vi "HFRR ADV v025 new software.vi"() -> ()   [LabVIEW 2025] (continued)
                        n2432 = Number To Fractional String(number=w3641, precision (6)=i16 2) -> (F-format string=w3642:string)  [unwired: 2 in]
                        n2433 = Concatenate Strings("Set Stroke [mm] :" ("Content"), w3642) -> (w3644:string)
                        n2434 = local read "EVENT LOG"() -> (w3646:string)
                        n2435 = call "Event Log.vi"("Content"=w3644, "EVENT LOG"=w3646) -> ("EVENT LOG"=w3645:string)  [unwired: 8 in, 1 out]
                        n2436 = local write "EVENT LOG"(w3645) -> ()
                      }
                      frame #26 {
                        n2437 = Wait (ms)(milliseconds to wait=u32 50) -> ()  [unwired: 1 out]
                      }
                      frame #27 {
                        n2438 = local read "Set Temp"() -> (w3649:dbl)
                        n2439 = Number To Fractional String(number=w3649, precision (6)=i16 2) -> (F-format string=w3650:string)  [unwired: 2 in]
                        n2440 = Concatenate Strings("Set Temperature [deg C] :" ("Content"), w3650) -> (w3652:string)
                        n2441 = local read "EVENT LOG"() -> (w3654:string)
                        n2442 = call "Event Log.vi"("Content"=w3652, "EVENT LOG"=w3654) -> ("EVENT LOG"=w3653:string)  [unwired: 8 in, 1 out]
                        n2443 = local write "EVENT LOG"(w3653) -> ()
                      }
                      frame #28 {
                        n2444 = Wait (ms)(milliseconds to wait=u32 50) -> ()  [unwired: 1 out]
                      }
                      frame #29 {
                        n2445 = local read "Set Rh"() -> (w3657:dbl)
                        n2446 = Number To Fractional String(number=w3657, precision (6)=i16 2) -> (F-format string=w3658:string)  [unwired: 2 in]
                        n2447 = Concatenate Strings("Set Humidity [%RH] :" ("Content"), w3658) -> (w3660:string)
                        n2448 = local read "EVENT LOG"() -> (w3662:string)
                        n2449 = call "Event Log.vi"("Content"=w3660, "EVENT LOG"=w3662) -> ("EVENT LOG"=w3661:string)  [unwired: 8 in, 1 out]
                        n2450 = local write "EVENT LOG"(w3661) -> ()
                      }
                      frame #30 {
                        n2451 = Wait (ms)(milliseconds to wait=u32 50) -> ()  [unwired: 1 out]
                      }
                      frame #31 {
                        n2452 = local read "test time"() -> (w3665:dbl)
                        n2453 = Number To Fractional String(number=w3665, precision (6)=i16 1) -> (F-format string=w3666:string)  [unwired: 2 in]
                        n2454 = Concatenate Strings("Test Duration [mins] :" ("Content"), w3666) -> (w3668:string)
                        n2455 = local read "EVENT LOG"() -> (w3670:string)
                        n2456 = call "Event Log.vi"("Content"=w3668, "EVENT LOG"=w3670) -> ("EVENT LOG"=w3669:string)  [unwired: 8 in, 1 out]
                        n2457 = local write "EVENT LOG"(w3669) -> ()
                      }
                      frame #32 {
                        w3671 = dbl[] [] ("History Data")
                        w3672 = cluster{"y":dbl, dbl, "y":dbl}[] [] ("History Data")
                        w3673 = FALSE ("Visible")
                        n2458 = property on="Stroke ( mm )" class="WFChart (strict)"("History Data"=w3672) -> ()  [unwired: 2 in, 2 out]
                        n2459 = property on="Humidity ( %RH )" class="WFChart (strict)"("History Data"=w3671) -> ()  [unwired: 2 in, 2 out]
                        n2460 = property on="Temperature ( Deg C )" class="WFChart (strict)"("History Data"=w3671) -> ()  [unwired: 2 in, 2 out]
                        n2461 = property on="Electrical Contact Resistance ( % )" class="WFChart (strict)"("History Data"=w3671) -> ()  [unwired: 2 in, 2 out]
                        n2462 = property on="Coefficient of Friction" class="WFChart (strict)"("History Data"=w3671) -> ()  [unwired: 2 in, 2 out]
                        n2463 = property on="Frictional Force ( N )" class="WFChart (strict)"("History Data"=w3671) -> ()  [unwired: 2 in, 2 out]
                        n2464 = property on="Coefficient of Friction" class="WFChart (strict)"("History Data"=w3671) -> ()  [unwired: 2 in, 2 out]
                        n2465 = property on="Frictional Force ( N )" class="WFChart (strict)"("History Data"=w3671) -> ()  [unwired: 2 in, 2 out]
                        n2466 = property on="Electrical Contact Resistance ( % )" class="WFChart (strict)"("History Data"=w3671) -> ()  [unwired: 2 in, 2 out]
                        n2467 = property on="Humidity ( %RH )" class="WFChart (strict)"("History Data"=w3671) -> ()  [unwired: 2 in, 2 out]
                        n2468 = property on="Stroke ( mm )" class="WFChart (strict)"("History Data"=w3672) -> ()  [unwired: 2 in, 2 out]
                        n2469 = property on="Temperature ( Deg C )" class="WFChart (strict)"("History Data"=w3671) -> ()  [unwired: 2 in, 2 out]
                        n2470 = property on="Service Password Log" class="Str"("Visible"=w3673) -> ()  [unwired: 2 in, 2 out]
                        n2471 = property on="Password 3" class="Clust (strict)"("Visible"=w3673) -> ()  [unwired: 2 in, 2 out]
                      }
                    }
                    "TEST FILE NAM,E SAVED" <- TRUE ("TEST FILE NAM,E SAVED")
                  }
                }
              }
            }
          }
        }
        n2472 = case shown="True" w2970 {
          frame False {
            n2473 = local write "tfalg"(0.0 ("tfalg")) -> ()
          }
          frame True {
            n2474 = local read "tfalg"() -> (w3115:dbl)
            n2475 = Equal?(x=w3115, y=0.0) -> (x = y?=w3116:bool)
            n2476 = case shown="True" w3116 {
              frame False {
              }
              frame True {
                n2477 = local read "Total No. of Tests"() -> (w3119:dbl)
                n2478 = local write "tfalg"(1.0 ("tfalg")) -> ()
                n2479 = local write "acq 2"(FALSE ("acq 2")) -> ()
                n2480 = Wait (ms)(milliseconds to wait=u32 200) -> ()  [unwired: 1 out]
                n2481 = Increment(x=w3119) -> (x+1=w3118:dbl)
                n2482 = local write "Total No. of Tests"(w3118) -> ()
              }
            }
          }
        }
        n2483 = local write "Test \nStatus"(w2976) -> ()
        n2484 = local write "Save"(w2976) -> ()
        n2485 = local read "Main Tab"() -> (w2933:T2)
        n2486 = case shown="True" w2957 {
          tunnel: [FALSE ("RUN") TRUE ("RUN")] -> w2956
          tunnel: [_ 1] -> w2949
          frame False {
          }
          frame True {
          }
        }
        n2487 = In Range and Coerce(upper limit=w2964, x=w2937, lower limit=w2963) -> (In Range?=w2955:bool)  [unwired: 1 out]
        n2488 = In Range and Coerce(upper limit=w2961, x=w2936, lower limit=w2962) -> (In Range?=w2953:bool)  [unwired: 1 out]
        n2489 = case shown="True" w2969 {
          frame False {
            n2490 = local read "Rt 3"() -> (w3097:bool)
            n2491 = case shown="True" w3097 {
              frame False {
              }
              frame True {
                n2492 = local write "Rt 3"(FALSE ("Rt 3")) -> ()
                n2493 = local write "Json End Flg"(TRUE ("Upld AR 2")) -> ()
              }
            }
            "Rt" <- TRUE ("Rt")
            "Rt 2" <- FALSE ("Rt")
          }
          frame True {
            n2494 = local read "Rt"() -> (w3104:bool)
            n2495 = local write "Rt 2"(TRUE ("Rt 2")) -> ()
            n2496 = case shown="True" w3104 {
              frame False {
              }
              frame True {
                w3105 = TRUE ("Upld AR 2")
                n2497 = local write "Rt"(FALSE ("Rt")) -> ()
                n2498 = local write "Upld AR"(w3105) -> ()
                n2499 = local write "Json St Flg"(w3105) -> ()
              }
            }
            "Rt 3" <- TRUE ("Rt 3")
          }
        }
        n2500 = case shown="True" w2955 {
          tunnel: [FALSE ("RUN") TRUE ("RUN")] -> w2954
          tunnel: [_ 2] -> w2948
          frame False {
          }
          frame True {
          }
        }
        n2501 = case shown="True" w2953 {
          tunnel: [FALSE ("RUN") TRUE ("RUN")] -> w2952
          tunnel: [_ 3] -> w2947
          frame False {
          }
          frame True {
          }
        }
        n2502 = case shown="\"Acquire\"" w2933 {
          tunnel: w2935 -> [_ w3166]
          frame Default {
            w3165 = 0.0 ("output")
            n2503 = local write "PID-out"(w3165) -> ()
            n2504 = local write "Frequency ( Hz )"(w3165) -> ()
          }
          frame "Acquire" {
            n2505 = stacked-sequence {
              frame #0 {
                n2506 = local read "Auto Start Test"() -> (w3168:bool)
                n2507 = case shown="True" w3168 {
                  tunnel: "RUN" -> [w3189 w3192]
                  tunnel: [w3189 w3191] -> w3169
                  frame False {
                  }
                  frame True {
                    n2508 = local read "Auto Start Temp"() -> (w3190:bool)
                    n2509 = Or(x=w3192, y=w3190) -> (x .or. y?=w3191:bool)
                  }
                }
                n2510 = local read "clk"() -> (w3188:dbl)
                n2511 = local read "Save"() -> (w3184:bool)
                n2512 = Equal?(x=w3188, y=0.0) -> (x = y?=w3185:bool)
                n2513 = And(x=w3185, y=w3184) -> (x .and. y?=w3186:bool)
                n2514 = Not(x="Engage") -> (.not. x?=w3175:bool)
                n2515 = case shown="False" w3169 {
                  tunnel: [0.0 w3215] -> w3171
                  frame False {
                    (unwired) TRUE ("Visible")
                    n2516 = local read "Auto Start Test"() -> (w3196:bool)
                    n2517 = local write "Start Time"(TRUE ("Start Time")) -> ()
                    n2518 = property on="Stroke 2" class="DigNum (strict)"("Visible"=FALSE) -> ()  [unwired: 2 in, 2 out]
                    n2519 = case shown="False" w3196 {
                      frame False {
                        n2520 = property on="Heater Button" class="Bool (strict)"("DisabledEnum"=T17."Enabled" ("Disabled")) -> ()  [unwired: 2 in, 2 out]
                        n2521 = property on="Humidity" class="Bool (strict)"("DisabledEnum"=T17."Enabled" ("Disabled")) -> ()  [unwired: 2 in, 2 out]
                      }
                      frame True {
                      }
                    }
                    n2522 = case shown="False" "TestCompFlg" {
                      frame False {
                        n2523 = local read "StartFlg"() -> (w3204:bool)
                        n2524 = case shown="True" w3204 {
                          frame False {
                          }
                          frame True {
                            n2525 = stacked-sequence {
                              frame #0 {
                                n2526 = local read "EVENT LOG"() -> (w3208:string)
                                n2527 = call "Event Log.vi"("Content"="Test was interrupted", "EVENT LOG"=w3208) -> ("EVENT LOG"=w3209:string)  [unwired: 8 in, 1 out]
                                n2528 = local write "EVENT LOG"(w3209) -> ()
                                n2529 = property on="RUN" class="Bool (strict)"("Visible"=TRUE) -> ()  [unwired: 2 in, 2 out]
                                n2530 = property on="Auto Start Test" class="Bool (strict)"("Visible"=TRUE) -> ()  [unwired: 2 in, 2 out]
                              }
                              frame #1 {
                                w3211 = FALSE ("StartFlg")
                                n2531 = property on="Heater Button" class="Bool (strict)"("Val(Sgnl)"=FALSE ("Value (Signaling)")) -> ()  [unwired: 2 in, 2 out]
                                n2532 = local write "Heater Button"(w3211) -> ()
                                n2533 = local write "StartFlg"(w3211) -> ()
                                n2534 = local write "Humidity"(w3211) -> ()
                              }
                              frame #2 {
                                n2535 = local write "Due Write"("VC;0" ("Command")) -> ()
                              }
                              frame #3 {
                                n2536 = Wait (ms)(milliseconds to wait=u32 1500) -> ()  [unwired: 1 out]
                              }
                              frame #4 {
                                n2537 = local write "Due Write"("HE;0" ("Command")) -> ()
                              }
                            }
                          }
                        }
                      }
                      frame True {
                      }
                    }
                    n2538 = local write "String 14"("Test will autostart once parameters reach the set value." ("String 14")) -> ()
                  }
                  frame True {
                    (unwired) FALSE ("Visible")
                    n2539 = property on="Stroke 2" class="DigNum (strict)"("Visible"=TRUE) -> ()  [unwired: 2 in, 2 out]
                    n2540 = property on="STOP 2" class="Bool (strict)"("Disabled"=u8 2) -> ()  [unwired: 2 in, 2 out]
                    n2541 = local write "String 14"(" Running....." ("String 14")) -> ()
                    n2542 = property on="Heater Button" class="Bool (strict)"("DisabledEnum"=T17."Disabled and Grayed Out" ("Disabled")) -> ()  [unwired: 2 in, 2 out]
                    n2543 = property on="Humidity" class="Bool (strict)"("DisabledEnum"=T17."Disabled and Grayed Out" ("Disabled")) -> ()  [unwired: 2 in, 2 out]
                    n2544 = case shown="True" "Start Time" {
                      selector: "Start Time" -> [_ w3234]
                      frame False {
                      }
                      frame True {
                        n2545 = Not(x=w3234) -> (.not. x?=w3233:bool)
                        n2546 = local write "Start Time"(w3233) -> ()
                        n2547 = local read "EVENT LOG"() -> (w3235:string)
                        n2548 = call "Event Log.vi"("Content"="Test in progress", "EVENT LOG"=w3235) -> ("EVENT LOG"=w3237:string)  [unwired: 8 in, 1 out]
                        n2549 = local write "EVENT LOG"(w3237) -> ()
                      }
                    }
                    n2550 = disable-structure shown="Enabled" {
                      disable-tunnel: [w3226 w3232] -> w3215
                      frame Disabled {
                        n2551 = local read "Set Hz"() -> (w3229:dbl)
                        n2552 = call <vilib>:"Uniform White Noise Waveform.vi"() -> ("signal out"=w3228:waveform(dbl))  [unwired: 10 in, 1 out]
                        n2553 = Random Number (0-1)() -> (number: 0 to 1=w3225:dbl)
                        n2554 = Add(x=w3229, y=w3228) -> (x+y=w3227:waveform(dbl))
                        n2555 = Multiply(x=ext 0.01 ("y"), y=w3225) -> (x*y=w3223:ext)
                        n2556 = Multiply(x=w3227, y=w3223) -> (x*y=w3226:waveform(ext))
                      }
                      frame Enabled {
                        n2557 = call-poly <vilib>:"Random Number (Range).vi"("lower bound (0)"=49.89, "upper bound (100)"=50.8) -> ("number"=w3232:dbl)  [unwired: 9 in]
                      }
                    }
                    "StartFlg" <- TRUE ("StartFlg")
                  }
                }
                n2558 = case shown="True" w3186 {
                  frame False {
                  }
                  frame True {
                    n2559 = local write "clk"(10.0 ("clk")) -> ()
                    n2560 = Get Date/Time In Seconds() -> (seconds since 1Jan1904=w3240:timestamp)
                    n2561 = To Double Precision Float(number=w3240) -> (double precision float=w3238:dbl)
                    n2562 = local write "acq timer"(w3238) -> ()
                    n2563 = local write "act save time"(w3238) -> ()
                  }
                }
                n2564 = call "Elapsed Time"("Time Target (s)"="Countdown", "Reset"=w3175) -> ("Elapsed Time (s)"=w3180:dbl, "Time has Elapsed"=w3178:bool)  [unwired: 10 in, 6 out]
                "Countdown 2" <- w3180
                n2565 = Subtract(x=w3180, y=2.0) -> (x-y=w3183:dbl)
                n2566 = Less?(x=w3183, y="Countdown") -> (x < y?=w3181:bool)
                n2567 = And(x=w3181, y=w3178) -> (x .and. y?=w3177:bool)
                n2568 = case shown="True" w3177 {
                  frame False {
                  }
                  frame True {
                    (unwired) dbl[] [] ("History Data")
                    n2569 = local write "Engage"(FALSE ("Engage")) -> ()
                    n2570 = local write "RUN"(TRUE ("RUN")) -> ()
                    n2571 = local read "Humidity ( %RH )"() -> (→"Rh Before":dbl)
                  }
                }
                n2572 = local read "Test \nStatus"() -> (w3173:bool)
                n2573 = Select(t=w3171, s=w3173, f=0.0) -> (s? t:f=w3172:dbl)
                n2574 = local write "Frequency ( Hz )"(w3172) -> ()
              }
              frame #1 {
                w3263 = 1000000.0 ("x")
                # "HC;1/0\nST;VALUE"
                # "Elapsed time\ncof\nstroke\nAir temp\nTemp\nHumidity"
                # "acq timer\n\nact save time"
                # "convert to microseconds"
                n2575 = local read "COUNT"() -> (w3246:i32)
                n2576 = local read "Rate"() -> (w3259:dbl)
                n2577 = Divide(x=w3263, y=w3259) -> (x/y=w3264:dbl)
                n2578 = Greater Or Equal?(x=w3246, y=250) -> (x >= y?=w3245:bool)
                n2579 = Get Date/Time In Seconds() -> (seconds since 1Jan1904=w3266:timestamp)
                n2580 = case shown="True" w3245 {
                  frame False {
                    n2581 = local read "COUNT"() -> (w3267:i32)
                    n2582 = Increment(x=w3267) -> (x+1=w3268:i32)
                    n2583 = local write "COUNT"(w3268) -> ()
                  }
                  frame True {
                    n2584 = local write "COUNT"(0 ("COUNT")) -> ()
                  }
                }
                n2585 = local read "Samplingtime 2"() -> (w3244:dbl)
                n2586 = local read "act save time"() -> (w3261:dbl)
                n2587 = Divide(x=w3264, y=w3263) -> (x/y=w3262:dbl)
                n2588 = To Double Precision Float(number=w3266) -> (double precision float=w3255:dbl)
                n2589 = Add(x=w3261, y=w3244) -> (x+y=w3260:dbl)
                n2590 = local read "acq timer"() -> (w3265:dbl)
                n2591 = local read "COUNT"() -> (w3248:i32)
                n2592 = Greater Or Equal?(x=w3255, y=w3260) -> (x >= y?=w3243:bool)
                n2593 = Multiply(x=w3262, y=w3248) -> (x*y=w3254:dbl)
                n2594 = Subtract(x=w3255, y=w3265) -> (x-y=w3257:dbl)
                n2595 = local read "Save"() -> (w3258:bool)
                n2596 = Add(x=w3257, y=w3254) -> (x+y=w3241:dbl)
                "Elapsed time 3" <- w3241
                n2597 = And(x=w3243, y=w3258) -> (x .and. y?=w3256:bool)
                n2598 = Divide(x=w3241, y=60.0) -> (x/y=w3252:dbl)
                n2599 = local read "Test \nStatus"() -> (w3242:bool)
                n2600 = local read "clk"() -> (w3249:dbl)
                n2601 = Equal?(x=w3249, y=10.0) -> (x = y?=w3251:bool)
                n2602 = case shown="True" w3256 {
                  tunnel: w3255 -> [_ w3379]
                  tunnel: [FALSE ("Boolean 2") TRUE ("Boolean 2")] -> _
                  frame False {
                  }
                  frame True {
                    w3333 = ";" ("Substring")
                    # "Pid out/\nFreq response value"
                    n2603 = local write "act save time"(w3379) -> ()
                    n2604 = local read "FILE"() -> (w3327:string)
                    n2605 = call "file check.vi"("file name in"=w3327) -> ("error out"=w3330:errorcluster, "file name out"=w3325:string)  [unwired: 9 in]
                    n2606 = local read "LVDT STROKE"() -> (w3322:dbl)
                    n2607 = local read "Add up Stroke"() -> (w3320:dbl)
                    n2608 = call "FILE PATH CREATION.vi"("error in"=w3330, "FILE NAME :"=w3325) -> ("FILE OUT"=w3328:path)  [unwired: 8 in, 1 out]
                    n2609 = Concatenate Strings(w3325, ".dgf" ("Substring")) -> (w3329:string)
                    n2610 = Subtract(x=w3322, y=w3320) -> (x-y=w3321:dbl)
                    n2611 = Absolute Value(x=w3321) -> (abs(x)=w3319:dbl)
                    n2612 = local read "FF 2"() -> (→"Frictional Force ( N )" →"Frictional Force ( N )":dbl)
                    n2613 = Build Path(base path=w3328, name or relative path=w3329) -> (appended path=w3324:path)
                    n2614 = local read "COF 2"() -> (w3338:dbl)
                    "cof" <- w3338
                    "Coefficient of Friction" <- w3338
                    "COF 4" <- w3338
                    "Coefficient of Friction" <- w3338
                    n2615 = local read "TEMP"() -> (w3341:dbl)
                    "Temp" <- w3341
                    "Temperature ( Deg C )" <- w3341
                    n2616 = local read "Humidity ( %RH )"() -> (w3340:dbl)
                    "Humidity ( %RH )" <- w3340
                    "Humidity ( %RH )" <- w3340
                    n2617 = local read "Frequency ( Hz )"() -> (w3347:dbl)
                    n2618 = call <vilib>:"Mean PtByPt.vi"("x"=w3319, "sample length"="STROKE FILTER") -> ("mean"=w3318:dbl)  [unwired: 2 in, 1 out]
                    n2619 = local read "Elapsed time"() -> (w3372:dbl)
                    n2620 = local read "AIR TEMP"() -> (w3345:dbl)
                    n2621 = local read "PID-out"() -> (w3350:dbl)
                    n2622 = local write "Temperature ( Deg C )"(w3341) -> ()
                    n2623 = Number To Fractional String(number=w3318, width (-)=i16 9 ("precision (6)"), precision (6)=i16 6) -> (F-format string=w3365:string)  [unwired: 1 in]
                    n2624 = Number To Fractional String(number=w3345, width (-)=i16 9 ("precision (6)"), precision (6)=i16 3) -> (F-format string=w3364:string)  [unwired: 1 in]
                    n2625 = Number To Fractional String(number=w3341, width (-)=i16 9 ("precision (6)"), precision (6)=i16 3) -> (F-format string=w3361:string)  [unwired: 1 in]
                    n2626 = Number To Fractional String(number=w3340, width (-)=i16 9 ("precision (6)"), precision (6)=i16 3) -> (F-format string=w3358:string)  [unwired: 1 in]
                    n2627 = Number To Fractional String(number=0.0, width (-)=i16 9 ("precision (6)"), precision (6)=i16 3) -> (F-format string=w3355:string)  [unwired: 1 in]
                    n2628 = Number To Fractional String(number=w3350, width (-)=i16 9 ("precision (6)"), precision (6)=i16 3) -> (F-format string=w3351:string)  [unwired: 1 in]
                    n2629 = Number To Fractional String(number=w3347, width (-)=i16 9 ("precision (6)"), precision (6)=i16 3) -> (F-format string=w3346:string)  [unwired: 1 in]
                    n2630 = Number To Fractional String(number=w3338, width (-)=i16 9 ("precision (6)"), precision (6)=i16 6) -> (F-format string=w3373:string)  [unwired: 1 in]
                    n2631 = Number To Fractional String(number=w3372, width (-)=i16 14 ("precision (6)"), precision (6)=i16 3) -> (F-format string=w3374:string)  [unwired: 1 in]
                    n2632 = Bundle("y"=1.02, "mean"=w3318, "y"=0.98) -> (w3339:cluster{"y":dbl, "mean":dbl, "y":dbl})  [unwired: 1 in]
                    n2633 = Number To Fractional String(number="Ambient Humidity :", width (-)=i16 9 ("precision (6)"), precision (6)=i16 6) -> (F-format string=w3331:string)  [unwired: 1 in]
                    n2634 = local read "RUN"() -> (w3337:bool)
                    n2635 = case shown="True" w3337 {
                      tunnel: w3339 -> [_ w3384]
                      tunnel: w3318 -> [_ w3383]
                      tunnel: w3318 -> [_ w3381]
                      tunnel: w3318 -> [_ w3382]
                      frame False {
                      }
                      frame True {
                        "Stroke ( mm )" <- w3384
                        "Stroke ( mm )" <- w3384
                        "Stroke 4" <- w3383
                        "Stroke 3" <- w3381
                        "Stroke 2" <- w3382
                        "measured_stroke" <- w3381
                      }
                    }
                    n2636 = Concatenate Strings(w3374, w3333, w3373, w3333, w3365, w3333, w3364, w3333, w3361, w3333, w3358, w3333, w3355, w3333, w3351, w3333, w3346, w3333, w3331, "\r") -> (w3371:string)
                    n2637 = call <vilib>:"Write Characters To File.vi"("append to file? (new file:F)"=TRUE, "character string"=w3371, "file path (dialog if empty)"=w3324) -> ()  [unwired: 2 in, 1 out]
                    "refresh flag" <- TRUE ("refresh flag")
                  }
                }
                n2638 = case shown="True" w3242 {
                  tunnel: w3252 -> [_ w3278]
                  tunnel: w3257 -> [_ w3288]
                  tunnel: [0.0 w3284] -> _
                  tunnel: w3251 -> [_ w3283]
                  tunnel: [0.0 w3282] -> _
                  tunnel: w3241 -> [_ w3282]
                  tunnel: w3255 -> [w3271 _]
                  frame False {
                    n2639 = local write "acq timer"(w3271) -> ()
                    n2640 = local write "Test Duration Status"(0.0 ("Test Duration Status")) -> ()
                  }
                  frame True {
                    n2641 = local read "Set Hz"() -> (w3285:dbl)
                    n2642 = local write "Elapsed time"(w3278) -> ()
                    n2643 = local read "test time"() -> (w3277:dbl)
                    n2644 = Multiply(x=w3288, y=w3285) -> (x*y=w3287:dbl)
                    n2645 = case shown="False" w3283 {
                      tunnel: w3287 -> [w3289 _]
                      tunnel: [w3289 1.0] -> w3284
                      frame False {
                        n2646 = local write "Cycles elapsed"(w3289) -> ()
                      }
                      frame True {
                      }
                    }
                    n2647 = Greater?(x=w3278, y=w3277) -> (0:w3286:bool)
                    n2648 = Subtract(x=w3277, y=w3278) -> (x-y=w3276:dbl)
                    "time" <- w3276
                    n2649 = Multiply(x=w3276, y=60.0) -> (x*y=w3275:dbl)
                    n2650 = local write "Time Remaining"(w3275) -> ()
                    n2651 = local write "Remaining Time"(w3275) -> ()
                    n2652 = case shown="True" w3286 {
                      frame False {
                      }
                      frame True {
                        n2653 = stacked-sequence {
                          frame #0 {
                            w3294 = T17."Enabled" ("Disabled")
                            w3293 = FALSE ("TEST FILE NAM,E SAVED")
                            w3295 = "" ("FILE")
                            w3296 = TRUE ("Visible")
                            n2654 = local write "Humidity"(FALSE ("Humidity")) -> ()
                            n2655 = local write "RUN"(FALSE ("OK Button 2")) -> ()
                            n2656 = local write "Heater Button"(FALSE ("Heater Button")) -> ()
                            n2657 = local write "Auto Start Test"(FALSE ("Auto Start Test")) -> ()
                            n2658 = local write "TestCompFlg"(TRUE ("StpFlg")) -> ()
                            n2659 = local read "Humidity ( %RH )"() -> (→"Rh After":dbl)
                            n2660 = property on="STOP 2" class="Bool (strict)"("Disabled"=u8 0) -> ()  [unwired: 2 in, 2 out]
                            n2661 = local read "EVENT LOG"() -> (w3301:string)
                            n2662 = call "Event Log.vi"("Content"="Test Completed", "EVENT LOG"=w3301) -> ("EVENT LOG"=w3300:string)  [unwired: 8 in, 1 out]
                            n2663 = property on="RUN" class="Bool (strict)"("Visible"=w3296) -> ()  [unwired: 2 in, 2 out]
                            n2664 = property on="Auto Start Test" class="Bool (strict)"("Visible"=w3296) -> ()  [unwired: 2 in, 2 out]
                            n2665 = local write "Batch Ref Num :"(w3295) -> ()
                            n2666 = local write "FILE"(w3295) -> ()
                            n2667 = local write "EVENT LOG"(w3300) -> ()
                            n2668 = local write "TEST FILE NAM,E SAVED"(w3293) -> ()
                            n2669 = local write "Fuel Discription :"(w3295) -> ()
                            n2670 = local write "START TEMP"(w3293) -> ()
                            n2671 = local write "Remarks :"(w3295) -> ()
                            n2672 = local write "Main Dashboard Buttons"(T1."Imaging" ("Main Dashboard Buttons")) -> ()
                            n2673 = local write "Main Tab"(T2."Adv Scar" ("Main Tab")) -> ()
                            n2674 = property on="FRICVALZ 2" class="Bool (strict)"("DisabledEnum"=w3294) -> ()  [unwired: 2 in, 2 out]
                            n2675 = property on="FRICVALZ 3" class="Bool (strict)"("DisabledEnum"=w3294) -> ()  [unwired: 2 in, 2 out]
                            n2676 = property on="FRICVALZ 4" class="Bool (strict)"("DisabledEnum"=w3294) -> ()  [unwired: 2 in, 2 out]
                          }
                          frame #1 {
                            n2677 = Wait (ms)(milliseconds to wait=u32 1500) -> ()  [unwired: 1 out]
                          }
                          frame #2 {
                            n2678 = local write "Due Write"("VC;0") -> ()
                          }
                          frame #3 {
                            n2679 = Wait (ms)(milliseconds to wait=u32 1500) -> ()  [unwired: 1 out]
                          }
                          frame #4 {
                            n2680 = local write "Due Write"("VC;0") -> ()
                          }
                          frame #5 {
                            n2681 = Wait (ms)(milliseconds to wait=u32 1500) -> ()  [unwired: 1 out]
                          }
                          frame #6 {
                            n2682 = local write "Due Write"("ST;0") -> ()
                          }
                          frame #7 {
                            n2683 = local write "measured_stroke"(0.0 ("measured_stroke")) -> ()
                            n2684 = Wait (ms)(milliseconds to wait=u32 1500) -> ()  [unwired: 1 out]
                          }
                          frame #8 {
                            n2685 = local write "Due Write"("HE;0") -> ()
                          }
                        }
                      }
                    }
                    n2686 = Divide(x=w3278, y=w3277) -> (x/y=w3281:dbl)
                    n2687 = Multiply(x=w3281, y=100.0) -> (x*y=w3279:dbl)
                    n2688 = local write "Test Duration Status"(w3279) -> ()
                  }
                }
              }
              frame #2 {
                n2689 = case shown="True" "Heater Button" {
                  tunnel: [0.0 ("output") w3407] -> w3385
                  frame False {
                    w3388 = TRUE ("tmpchk")
                    n2690 = local read "TEMP"() -> (w3389:dbl)
                    n2691 = local write "Temp ini"(w3389) -> ()
                    n2692 = local write "Reset 4"(w3388) -> ()
                    n2693 = local write "tmpchk"(w3388) -> ()
                    n2694 = local write "reinit"(TRUE ("reinit")) -> ()
                    n2695 = local write "manual temp log"(TRUE ("manual temp log")) -> ()
                  }
                  frame True {
                    # "Logic to turn off\nthe heater when \ntemp is not rising.\nTime - 60 sec\nDelta t- 5°c"
                    n2696 = local read "Temp ini"() -> (w3396:dbl)
                    n2697 = local read "Auto Start Test"() -> (w3392:bool)
                    n2698 = Less?(x=w3396, y=53.0) -> (x < y?=w3394:bool)
                    n2699 = case shown="False" w3392 {
                      frame False {
                        n2700 = local read "Set Temp"() -> (w3416:dbl)
                        n2701 = local read "TEMP"() -> (w3415:dbl)
                        n2702 = Subtract(x=w3416, y=w3415) -> (x-y=w3414:dbl)
                        n2703 = Absolute Value(x=w3414) -> (abs(x)=w3413:dbl)
                        n2704 = Less?(x=w3413, y=0.5) -> (x < y?=w3411:bool)
                        n2705 = case shown="True" w3411 {
                          tunnel: "manual temp log" -> [_ w3417]
                          frame False {
                          }
                          frame True {
                            n2706 = case shown="True" w3417 {
                              selector: w3417 -> [_ w3418]
                              frame False {
                              }
                              frame True {
                                # "#Event log"
                                n2707 = Not(x=w3418) -> (.not. x?=w3419:bool)
                                n2708 = local write "manual temp log"(w3419) -> ()
                                n2709 = local read "EVENT LOG"() -> (w3422:string)
                                n2710 = call "Event Log.vi"("Content"="Target Temperature reached", "EVENT LOG"=w3422) -> ("EVENT LOG"=w3421:string)  [unwired: 8 in, 1 out]
                                n2711 = local write "EVENT LOG"(w3421) -> ()
                              }
                            }
                          }
                        }
                      }
                      frame True {
                        n2712 = local write "manual temp log"(TRUE ("manual temp log")) -> ()
                      }
                    }
                    n2713 = And(x="tmpchk", y=w3394) -> (x .and. y?=w3397:bool)
                    n2714 = case shown="True" w3397 {
                      frame False {
                      }
                      frame True {
                        n2715 = call "Elapsed Time8"("Time Target (s)"=300.0, "Reset"="Reset 4") -> ("Time has Elapsed"=w3424:bool)  [unwired: 10 in, 7 out]
                        n2716 = flat-sequence {
                          tunnel: w3424 -> [_]
                          frame #0 {
                            n2717 = local write "Reset 4"(FALSE ("Reset 4")) -> ()
                          }
                        }
                        n2718 = case shown="True" w3424 {
                          frame False {
                          }
                          frame True {
                            n2719 = local read "Temp ini"() -> (w3431:dbl)
                            n2720 = Add(x=w3431, y=5.0) -> (x+y=w3429:dbl)
                            n2721 = local read "TEMP"() -> (w3432:dbl)
                            n2722 = Greater?(x=w3432, y=w3429) -> (0:w3430:bool)
                            n2723 = case shown="False" w3430 {
                              frame False {
                                n2724 = local write "Heater Button"(FALSE ("Heater Button")) -> ()
                              }
                              frame True {
                                n2725 = local write "tmpchk"(FALSE ("tmpchk")) -> ()
                              }
                            }
                          }
                        }
                      }
                    }
                    n2726 = local read "Set Temp"() -> (w3405:dbl)
                    n2727 = local read "TEMP"() -> (w3399:dbl)
                    n2728 = call-poly <vilib>:"PID.vi"("reinitialize? (F)"="reinit", "dt (s)"=-1.0, "process variable"=w3399, "setpoint"=w3405) -> ("output"=w3402:dbl)  [unwired: 6 in, 1 out]
                    n2729 = Subtract(x=w3405, y=w3399) -> (x-y=w3406:dbl)
                    n2730 = Add(x=w3405, y=0.5) -> (x+y=w3403:dbl)
                    n2731 = Greater Or Equal?(x=w3399, y=w3403) -> ()  [unwired: 1 out]
                    n2732 = Select(t=0.0, s=FALSE, f=w3402) -> (s? t:f=w3401:dbl)
                    "PID output" <- w3401
                    n2733 = flat-sequence {
                      tunnel: w3401 -> [w3435]
                      tunnel: [w3435] -> w3407
                      frame #0 {
                        n2734 = local write "reinit"(FALSE ("reinit")) -> ()
                      }
                    }
                    n2735 = Bundle(w3406, "output"=w3401, "TEMP"=w3399) -> ()  [unwired: 1 in, 1 out]
                  }
                }
                "PID-out" <- w3385
              }
              frame #3 {
                n2736 = local read "TEMP"() -> (w3437:dbl)
                n2737 = Greater Or Equal?(x=w3437, y="Set Temp 2") -> (x >= y?=w3442:bool)
                n2738 = case shown="True" w3442 {
                  tunnel: [FALSE TRUE] -> w3440
                  frame False {
                  }
                  frame True {
                  }
                }
                "Status 13" <- w3440
                n2739 = And(x=w3440, y="trip1 8") -> (x .and. y?=w3439:bool)
                n2740 = case shown="True" w3439 {
                  frame False {
                    n2741 = local write "Heater Trip Temp"(TRUE ("Heater Trip Temp")) -> ()
                  }
                  frame True {
                    w3445 = FALSE ("OK Button 2")
                    n2742 = case shown="True" "Heater Trip Temp" {
                      selector: "Heater Trip Temp" -> [_ w3447]
                      frame False {
                      }
                      frame True {
                        n2743 = Not(x=w3447) -> (.not. x?=w3446:bool)
                        n2744 = local read "EVENT LOG"() -> (w3450:string)
                        n2745 = local write "Heater Trip Temp"(w3446) -> ()
                        n2746 = call "Event Log.vi"("Content"="Heater Trip", "EVENT LOG"=w3450) -> ("EVENT LOG"=w3449:string)  [unwired: 8 in, 1 out]
                        n2747 = local write "EVENT LOG"(w3449) -> ()
                      }
                    }
                    n2748 = local write "RUN"(w3445) -> ()
                    n2749 = property on="Auto Start Test" class="Bool (strict)"("Value"=w3445) -> ()  [unwired: 2 in, 2 out]
                    n2750 = local write "Heater Button"(w3445) -> ()
                  }
                }
              }
            }
            n2751 = case shown="False" w3166 {
              frame False {
                n2752 = disable-structure shown="Disabled" {
                  frame Disabled {
                    n2753 = stacked-sequence {
                      frame #0 {
                        n2754 = local write "RUN"(FALSE ("OK Button 2")) -> ()
                      }
                      frame #1 {
                      }
                    }
                  }
                  frame Enabled {
                  }
                }
              }
              frame True {
              }
            }
          }
        }
        n2755 = local read "airtempflg"() -> (w2958:bool)
        n2756 = Or(x=w2958, y=w2956) -> (x .or. y?=w2959:bool)
        n2757 = Insert Into Array(array=string[] ["Air Temperature has reached set value,", "Humidity has reached set value,", "Sample Temperaturehas reached set value,", ""], index=0, new element="") -> (w2944:string[])
        n2758 = Build Array(w2949, w2948, w2947) -> (w2945:i32[])
        n2759 = disable-structure shown="Disabled" {
          disable-tunnel: w2959 -> [w3036 _]
          disable-tunnel: w2954 -> [w3035 _]
          disable-tunnel: w2952 -> [w3034 _]
          frame Disabled {
            n2760 = Compound Arithmetic op=AND(w3036, w3035, w3034) -> ()  [unwired: 1 out]
            n2761 = case shown="True" {
              selector: _ -> [_ _]
              frame False {
              }
              frame True {
                w3037 = FALSE ("autostrtflg")
                n2762 = local write "RUN"(TRUE ("RUN")) -> ()
                n2763 = local write "autostrtflg"(w3037) -> ()
                n2764 = local write "autostart"(w3037) -> ()
                n2765 = local write "String 14"(" Running....." ("String 14")) -> ()
              }
            }
          }
          frame Enabled {
          }
        }
        n2766 = for {
          tunnel: w2945 -> [w3087] mode=indexing
          tunnel: w2944 -> [w3086]
          shift-right: [w3083] -> w2943
          shift-left: "" -> [w3085]
          n2767 = Index Array(array=w3086, index=w3087) -> (element=w3084:string)
          n2768 = Concatenate Strings(w3084, w3085) -> (w3083:string)
        }
        n2769 = local write "autostart 2"(w2943) -> ()
        n2770 = local read "Reset Graph"() -> (w2932:bool)
        n2771 = case shown="True" w2932 {
          selector: w2932 -> [_ w2986]
          frame False {
          }
          frame True {
            w3000 = 0.0 ("X Scale.Range:Maximum")
            n2772 = Not(x=w2986) -> (.not. x?=w2985:bool)
            n2773 = local write "Reset Graph"(w2985) -> ()
            n2774 = property on="Electrical Contact Resistance ( % )" class="WFChart (strict)"("XScale.Maximum"=600.0 ("X Scale.Range:Maximum"), "XScale.Minimum"=0.0 ("X Scale.Range:Minimum"), "YScale.Maximum"=100.0 ("Y Scale.Range:Maximum"), "YScale.Minimum"=0.0 ("Y Scale.Range:Minimum")) -> ()  [unwired: 2 in, 2 out]
            n2775 = property on="Frictional Force ( N )" class="WFChart (strict)"("XScale.Maximum"=600.0 ("X Scale.Range:Maximum"), "XScale.Minimum"=0.0 ("X Scale.Range:Minimum"), "YScale.Maximum"=100.0 ("Y Scale.Range:Maximum"), "YScale.Minimum"=0.0 ("Y Scale.Range:Minimum")) -> ()  [unwired: 2 in, 2 out]
            n2776 = property on="Temperature ( Deg C )" class="WFChart (strict)"("XScale.Maximum"=600.0 ("X Scale.Range:Maximum"), "XScale.Minimum"=0.0 ("X Scale.Range:Minimum"), "YScale.Maximum"=100.0 ("Y Scale.Range:Maximum"), "YScale.Minimum"=0.0 ("Y Scale.Range:Minimum")) -> ()  [unwired: 2 in, 2 out]
            n2777 = property on="Humidity ( %RH )" class="WFChart (strict)"("XScale.Maximum"=600.0 ("X Scale.Range:Maximum"), "XScale.Minimum"=0.0 ("X Scale.Range:Minimum"), "YScale.Maximum"=100.0 ("Y Scale.Range:Maximum"), "YScale.Minimum"=0.0 ("Y Scale.Range:Minimum")) -> ()  [unwired: 2 in, 2 out]
            n2778 = property on="Stroke ( mm )" class="WFChart (strict)"("XScale.Maximum"=600.0 ("X Scale.Range:Maximum"), "XScale.Minimum"=0.0 ("X Scale.Range:Minimum"), "YScale.Maximum"=100.0 ("Y Scale.Range:Maximum"), "YScale.Minimum"=0.0 ("Y Scale.Range:Minimum")) -> ()  [unwired: 2 in, 2 out]
            n2779 = property on="Coefficient of Friction" class="WFChart (strict)"("XScale.Maximum"=600.0 ("X Scale.Range:Maximum"), "XScale.Minimum"=0.0 ("X Scale.Range:Minimum"), "YScale.Maximum"=100.0 ("Y Scale.Range:Maximum"), "YScale.Minimum"=0.0 ("Y Scale.Range:Minimum")) -> ()  [unwired: 2 in, 2 out]
            n2780 = property on="Electrical Contact Resistance ( % )" class="WFChart (strict)"("XScale.Minimum"=0.0 ("X Scale.Range:Minimum"), "XScale.Maximum"=600.0 ("X Scale.Range:Maximum"), "YScale.Minimum"=0.0 ("Y Scale.Range:Minimum"), "YScale.Maximum"=100.0 ("Y Scale.Range:Maximum")) -> ()  [unwired: 2 in, 2 out]
            n2781 = property on="Temperature ( Deg C )" class="WFChart (strict)"("XScale.Minimum"=0.0 ("X Scale.Range:Minimum"), "XScale.Maximum"=600.0 ("X Scale.Range:Maximum"), "YScale.Minimum"=0.0 ("Y Scale.Range:Minimum"), "YScale.Maximum"=100.0 ("Y Scale.Range:Maximum")) -> ()  [unwired: 2 in, 2 out]
            n2782 = property on="Coefficient of Friction" class="WFChart (strict)"("XScale.Minimum"=0.0 ("X Scale.Range:Minimum"), "XScale.Maximum"=600.0 ("X Scale.Range:Maximum"), "YScale.Maximum"=1.0 ("X Scale.Range:Minimum"), "YScale.Minimum"=0.0 ("X Scale.Range:Minimum")) -> ()  [unwired: 2 in, 2 out]
            n2783 = property on="Frictional Force ( N )" class="WFChart (strict)"("XScale.Maximum"=600.0 ("X Scale.Range:Maximum"), "XScale.Minimum"=w3000, "YScale.Maximum"=10.0 ("Y Scale.Range:Maximum"), "YScale.Minimum"=w3000) -> ()  [unwired: 2 in, 2 out]
            n2784 = property on="Stroke ( mm )" class="WFChart (strict)"("XScale.Maximum"=600.0 ("X Scale.Range:Maximum"), "XScale.Minimum"=0.0 ("X Scale.Range:Minimum"), "YScale.Maximum"=100.0 ("Y Scale.Range:Maximum"), "YScale.Minimum"=0.0 ("Y Scale.Range:Minimum")) -> ()  [unwired: 2 in, 2 out]
            n2785 = property on="Humidity ( %RH )" class="WFChart (strict)"("XScale.Maximum"=600.0 ("X Scale.Range:Maximum"), "XScale.Minimum"=0.0 ("X Scale.Range:Minimum"), "YScale.Maximum"=100.0 ("Y Scale.Range:Maximum"), "YScale.Minimum"=0.0 ("Y Scale.Range:Minimum")) -> ()  [unwired: 2 in, 2 out]
          }
        }
      }
      frame "Compare Files" {
        # "Elapsed time\ncof\nstroke\nAir temp\nTemp\nHumidity"
        n2786 = case shown="True" "RSTV1 2" {
          frame False {
          }
          frame True {
            n2787 = property on="Humidity ( %RH )" class="XYGraph (strict)"("Y Scale.Display Format:Precision"=u8 0 ("Y Scale.Format & Precision:Precision")) -> ()  [unwired: 2 in, 2 out]
            n2788 = property on="Humidity ( %RH )" class="XYGraph (strict)"("X Scale.Range:Minimum"=0.0, "X Scale.Range:Maximum"=75.0, "Y Scale.Range:Minimum"=48.0, "Y Scale.Range:Maximum"=58.0) -> ()  [unwired: 2 in, 2 out]
          }
        }
        n2789 = case shown="True" "RST CP 2" {
          frame False {
          }
          frame True {
            n2790 = property on="XY Graph 13" class="XYGraph (strict)"("Y Scale.Display Format:Precision"=u8 0 ("Y Scale.Format & Precision:Precision")) -> ()  [unwired: 2 in, 2 out]
            n2791 = property on="XY Graph 13" class="XYGraph (strict)"("X Scale.Range:Minimum"=0.0, "X Scale.Range:Maximum"=75.0, "Y Scale.Range:Minimum"=0.0, "Y Scale.Range:Maximum"=100.0) -> ()  [unwired: 2 in, 2 out]
          }
        }
        n2792 = case shown="True" "RST CP" {
          frame False {
          }
          frame True {
            n2793 = property on="Sample Temperature ( °C )" class="XYGraph (strict)"("Y Scale.Display Format:Precision"=u8 2 ("Y Scale.Format & Precision:Precision")) -> ()  [unwired: 2 in, 2 out]
            n2794 = property on="Sample Temperature ( °C )" class="XYGraph (strict)"("X Scale.Range:Minimum"=0.0, "X Scale.Range:Maximum"=75.0, "Y Scale.Range:Minimum"=58.0, "Y Scale.Range:Maximum"=62.0) -> ()  [unwired: 2 in, 2 out]
          }
        }
        n2795 = case shown="True" "RSTV1 3" {
          frame False {
          }
          frame True {
            n2796 = property on="Air Temperature  ( °C )" class="XYGraph (strict)"("Y Scale.Display Format:Precision"=u8 2 ("Y Scale.Format & Precision:Precision")) -> ()  [unwired: 2 in, 2 out]
            n2797 = property on="Air Temperature  ( °C )" class="XYGraph (strict)"("X Scale.Range:Minimum"=0.0 ("Y Scale.Range:Minimum"), "X Scale.Range:Maximum"=75.0 ("Y Scale.Range:Maximum"), "Y Scale.Range:Minimum"=20.0 ("X Scale.Range:Minimum"), "Y Scale.Range:Maximum"=26.0 ("X Scale.Range:Maximum")) -> ()  [unwired: 2 in, 2 out]
          }
        }
        n2798 = case shown="True" "RSTV1 4" {
          frame False {
          }
          frame True {
            n2799 = property on="Stroke ( mm )" class="XYGraph (strict)"("Y Scale.Display Format:Precision"=u8 2 ("Y Scale.Format & Precision:Precision")) -> ()  [unwired: 2 in, 2 out]
            n2800 = property on="Stroke ( mm )" class="XYGraph (strict)"("X Scale.Range:Minimum"=0.0 ("Y Scale.Range:Maximum"), "X Scale.Range:Maximum"=75.0 ("X Scale.Range:Minimum"), "Y Scale.Range:Minimum"=0.98, "Y Scale.Range:Maximum"=1.02) -> ()  [unwired: 2 in, 2 out]
          }
        }
        n2801 = case shown="True" "rstv2" {
          frame False {
          }
          frame True {
            n2802 = property on="Coefficient Of Friction" class="XYGraph (strict)"("Y Scale.Display Format:Precision"=u8 3 ("Y Scale.Format & Precision:Precision")) -> ()  [unwired: 2 in, 2 out]
            n2803 = property on="Coefficient Of Friction" class="XYGraph (strict)"("X Scale.Range:Minimum"=0.0 ("Y Scale.Range:Maximum"), "X Scale.Range:Maximum"=75.0, "Y Scale.Range:Minimum"=0.0, "Y Scale.Range:Maximum"=1.0 ("X Scale.Range:Minimum")) -> ()  [unwired: 2 in, 2 out]
          }
        }
        n2804 = case shown="True" "RST CP 3" {
          frame False {
          }
          frame True {
            n2805 = property on="Air Temp ( °C ) vs Humidity ( % RH )" class="XYGraph (strict)"("X Scale.Range:Minimum"=18.0, "X Scale.Range:Maximum"=28.0 ("X Scale.Range:Minimum"), "Y Scale.Range:Minimum"=30.0 ("X Scale.Range:Minimum"), "Y Scale.Range:Maximum"=70.0 ("X Scale.Range:Minimum")) -> ()  [unwired: 2 in, 2 out]
          }
        }
        n2806 = case shown="True" "OPEN 1" {
          frame False {
          }
          frame True {
            (unwired) 0  # existing file
            w3726 = "Choose a datalog file to open"  # prompt
            n2807 = local write "OPEN 1"(FALSE ("OPEN 1")) -> ()
            n2808 = String To Path(string="C:\\LAB-IQ\\Data\\") -> (path=w3711:path)
            n2809 = File Dialog(6:"*.dgf" ("pattern"), 7:w3726, 11:w3711) -> (0:w3709:errorcluster, 3:w3717:path)  [unwired: 4 in, 2 out]
            n2810 = Unbundle(w3709) -> ()  [unwired: 3 out]
            n2811 = Strip Path(path=w3717) -> (name=w3716:string)  [unwired: 1 out]
            n2812 = Path To String(path=w3717) -> (string=w3712:string)
            "string1" <- w3712
            n2813 = Match Pattern(string=w3716, regular expression=".dgf") -> (before substring=→"String Control":string)  [unwired: 1 in, 3 out]
            n2814 = Match Pattern(string=w3712, regular expression=".dgf" ("substring (\"\")")) -> (before substring=w3722:string)  [unwired: 1 in, 3 out]
            n2815 = Concatenate Strings(w3722, ".duf" ("Substring")) -> (w3718:string)
            n2816 = String To Path(string=w3718) -> (path=w3723:path)
            n2817 = call <vilib>:"Read Characters From File.vi"("file path (dialog if empty)"=w3723, "start of read offset (chars.:0)"=60 ("start of read offset (chars.: 0)")) -> ("character string"=→"String Control 2":string)  [unwired: 4 in, 3 out]
          }
        }
        n2818 = case shown="True" "OPEN 2" {
          frame False {
          }
          frame True {
            (unwired) 0  # existing file
            w3744 = "Choose a datalog file to open"  # prompt
            n2819 = local write "OPEN 2"(FALSE ("OPEN 1")) -> ()
            n2820 = String To Path(string="C:\\LAB-IQ\\Data\\") -> (path=w3729:path)
            n2821 = File Dialog(6:"*.dgf" ("pattern"), 7:w3744, 11:w3729) -> (0:w3727:errorcluster, 3:w3735:path)  [unwired: 4 in, 2 out]
            n2822 = Unbundle(w3727) -> ()  [unwired: 3 out]
            n2823 = Strip Path(path=w3735) -> (name=w3733:string)  [unwired: 1 out]
            n2824 = Path To String(path=w3735) -> (string=w3730:string)
            "string1 2" <- w3730
            n2825 = Match Pattern(string=w3733, regular expression=".dgf") -> (before substring=→"String Control 3":string)  [unwired: 1 in, 3 out]
            n2826 = Match Pattern(string=w3730, regular expression=".dgf" ("substring (\"\")")) -> (before substring=w3741:string)  [unwired: 1 in, 3 out]
            n2827 = Concatenate Strings(w3741, ".duf" ("Substring")) -> (w3738:string)
            n2828 = String To Path(string=w3738) -> (path=w3736:path)
            n2829 = call <vilib>:"Read Characters From File.vi"("file path (dialog if empty)"=w3736, "start of read offset (chars.:0)"=60 ("start of read offset (chars.: 0)")) -> ("character string"=→"String Control 4":string)  [unwired: 4 in, 3 out]
          }
        }
        n2830 = case shown="True" "OPEN 3" {
          frame False {
          }
          frame True {
            (unwired) 0  # existing file
            w3762 = "Choose a datalog file to open"  # prompt
            n2831 = local write "OPEN 3"(FALSE ("OPEN 1")) -> ()
            n2832 = String To Path(string="C:\\LAB-IQ\\Data\\") -> (path=w3747:path)
            n2833 = File Dialog(6:"*.dgf" ("pattern"), 7:w3762, 11:w3747) -> (0:w3745:errorcluster, 3:w3753:path)  [unwired: 4 in, 2 out]
            n2834 = Unbundle(w3745) -> ()  [unwired: 3 out]
            n2835 = Strip Path(path=w3753) -> (name=w3751:string)  [unwired: 1 out]
            n2836 = Path To String(path=w3753) -> (string=w3748:string)
            "string1 3" <- w3748
            n2837 = Match Pattern(string=w3751, regular expression=".dgf") -> (before substring=→"String Control 5":string)  [unwired: 1 in, 3 out]
            n2838 = Match Pattern(string=w3748, regular expression=".dgf" ("substring (\"\")")) -> (before substring=w3758:string)  [unwired: 1 in, 3 out]
            n2839 = Concatenate Strings(w3758, ".duf" ("Substring")) -> (w3755:string)
            n2840 = String To Path(string=w3755) -> (path=w3759:path)
            n2841 = call <vilib>:"Read Characters From File.vi"("file path (dialog if empty)"=w3759, "start of read offset (chars.:0)"=60 ("start of read offset (chars.: 0)")) -> ("character string"=→"String Control 6":string)  [unwired: 4 in, 3 out]
          }
        }
        n2842 = case shown="True" "OPEN 4" {
          frame False {
          }
          frame True {
            (unwired) 0  # existing file
            w3780 = "Choose a datalog file to open"  # prompt
            n2843 = local write "OPEN 4"(FALSE ("OPEN 1")) -> ()
            n2844 = String To Path(string="C:\\LAB-IQ\\Data\\") -> (path=w3765:path)
            n2845 = File Dialog(6:"*.dgf" ("pattern"), 7:w3780, 11:w3765) -> (0:w3763:errorcluster, 3:w3771:path)  [unwired: 4 in, 2 out]
            n2846 = Unbundle(w3763) -> ()  [unwired: 3 out]
            n2847 = Strip Path(path=w3771) -> (name=w3769:string)  [unwired: 1 out]
            n2848 = Path To String(path=w3771) -> (string=w3766:string)
            "string1 4" <- w3766
            n2849 = Match Pattern(string=w3769, regular expression=".dgf") -> (before substring=→"String Control 7":string)  [unwired: 1 in, 3 out]
            n2850 = Match Pattern(string=w3766, regular expression=".dgf" ("substring (\"\")")) -> (before substring=w3776:string)  [unwired: 1 in, 3 out]
            n2851 = Concatenate Strings(w3776, ".duf" ("Substring")) -> (w3773:string)
            n2852 = String To Path(string=w3773) -> (path=w3777:path)
            n2853 = call <vilib>:"Read Characters From File.vi"("file path (dialog if empty)"=w3777, "start of read offset (chars.:0)"=60 ("start of read offset (chars.: 0)")) -> ("character string"=→"String Control 8":string)  [unwired: 4 in, 3 out]
          }
        }
      }
      frame "About" {
        # "Elapsed time\ncof\nstroke\nmean pos\nTemp\nHumidity"
        n2854 = disable-structure shown="Disabled" {
          frame Disabled {
            n2855 = case shown="True" "Export" {
              frame False {
              }
              frame True {
                w3802 = "                                      " ("string")
                w3804 = "\r"
                (unwired) i16 6 ("width (-)")
                w3881 = "\r"
                w3813 = "\r"
                n2856 = local write "Export"(FALSE ("Export")) -> ()
                n2857 = local read "String 29"() -> (w3850:string)
                n2858 = local read "String 34"() -> (w3838:string)
                n2859 = local read "String 35"() -> (w3833:string)
                n2860 = local read "String 37"() -> (w3829:string)
                n2861 = local read "String 36"() -> (w3826:string)
                n2862 = local read "String 38"() -> (w3823:string)
                n2863 = local read "String 39"() -> (w3820:string)
                n2864 = Match Pattern(string=w3850, regular expression=".dwm") -> (before substring=w3846:string)  [unwired: 1 in, 3 out]
                "before substring" <- w3846
                n2865 = local read "S 38"() -> (w3841:string)
                n2866 = local read "S 39"() -> (w3834:string)
                n2867 = local read "Temperature before test 2"() -> (w3870:dbl)
                n2868 = local read "Temperature after test 2"() -> (w3875:dbl)
                n2869 = local read "Humidity before test 2"() -> (w3856:dbl)
                n2870 = local read "Humidity after test 2"() -> (w3871:dbl)
                n2871 = local read "MWSD 2"() -> (w3867:dbl)
                n2872 = local read "WS1.4 2"() -> (w3883:dbl)
                n2873 = local read "HCF 2"() -> (w3879:dbl)
                n2874 = local read "AVP 2"() -> (w3868:dbl)
                n2875 = Concatenate Strings("1," ("string"), w3841) -> (w3840:string)
                n2876 = Concatenate Strings("2," ("string"), w3838) -> (w3837:string)
                n2877 = Concatenate Strings("3," ("string"), w3834) -> (w3836:string)
                n2878 = Concatenate Strings("4," ("string"), w3833) -> (w3832:string)
                n2879 = Concatenate Strings("5," ("string"), w3829) -> (w3830:string)
                n2880 = Concatenate Strings("6," ("string"), w3826) -> (w3827:string)
                n2881 = Concatenate Strings("7," ("string"), w3823) -> (w3824:string)
                n2882 = Concatenate Strings("8," ("string"), w3820) -> (w3821:string)
                n2883 = local read "Sample ID"() -> (w3888:string)
                n2884 = case shown="\"xlx\"" "Select File Type" {
                  tunnel: w3846 -> [w3891 w3893 w3895]
                  tunnel: [w3889 w3894 w3896] -> w3845
                  frame "xlx" {
                    n2885 = Concatenate Strings(w3891, ".xls" ("string")) -> (w3889:string)
                  }
                  frame "csv" {
                    n2886 = Concatenate Strings(w3893, ".csv" ("string")) -> (w3894:string)
                  }
                  frame "txt" {
                    n2887 = Concatenate Strings(w3895, ".txt" ("string")) -> (w3896:string)
                  }
                }
                n2888 = local read "Test Date"() -> (w3887:string)
                n2889 = local read "String 45"() -> (w3801:string)
                n2890 = local read "String 31"() -> (w3886:string)
                n2891 = local read "String 32"() -> (w3885:string)
                n2892 = local read "TITTLE"() -> (w3809:string)
                n2893 = Number To Fractional String(number=w3856, width (-)=i16 6, precision (6)=i16 2) -> (F-format string=w3855:string)  [unwired: 1 in]
                n2894 = Number To Fractional String(number=w3870, width (-)=i16 6, precision (6)=i16 2) -> (F-format string=w3876:string)  [unwired: 1 in]
                n2895 = Number To Fractional String(number=w3871, width (-)=i16 6, precision (6)=i16 2) -> (F-format string=w3869:string)  [unwired: 1 in]
                n2896 = Number To Fractional String(number=w3875, width (-)=i16 6, precision (6)=i16 2) -> (F-format string=w3874:string)  [unwired: 1 in]
                n2897 = Number To Fractional String(number=w3867, width (-)=i16 6, precision (6)=i16 2) -> (F-format string=w3865:string)  [unwired: 1 in]
                n2898 = Number To Fractional String(number=w3868, width (-)=i16 6, precision (6)=i16 2) -> (F-format string=w3866:string)  [unwired: 1 in]
                n2899 = Number To Fractional String(number=w3879, width (-)=i16 6, precision (6)=i16 2) -> (F-format string=w3880:string)  [unwired: 1 in]
                n2900 = Number To Fractional String(number=w3883, precision (6)=i16 2) -> (F-format string=w3884:string)  [unwired: 2 in]
                n2901 = local read "s.NO"() -> (w3803:string)
                n2902 = Concatenate Strings("=" ("string"), w3809) -> (w3808:string)
                n2903 = Concatenate Strings("S.No," ("string"), "                                       Parameters" ("string")) -> (w3814:string)
                n2904 = Concatenate Strings(w3881, w3840, w3855, w3881, w3837, w3876, w3881, w3836, w3869, w3881, w3832, w3874, w3881, w3830, w3865, w3881, w3827, w3866, w3881, w3824, w3880, w3881, w3821, w3884) -> (w3843:string)
                n2905 = Concatenate Strings(w3813, "," ("string"), w3801, w3803, w3802, w3885, w3888, w3802, w3886, w3887, w3813) -> (w3811:string)
                n2906 = local read "Tested by"() -> (w3817:string)
                n2907 = local read "String 33"() -> (w3818:string)
                n2908 = Concatenate Strings("," ("string"), "                                                                             " ("string")) -> (w3806:string)
                n2909 = Concatenate Strings(w3808, w3804, w3811, w3804, w3814, w3843, w3804, w3806, w3818, w3817) -> (→"export":string)
                n2910 = String To Path(string=w3845) -> (path=w3852:path)
                n2911 = local read "export"() -> (w3847:string)
                n2912 = call <vilib>:"Write Characters To File.vi"("append to file? (new file:F)"=FALSE, "character string"=w3847, "file path (dialog if empty)"=w3852) -> ()  [unwired: 2 in, 1 out]
              }
            }
          }
          frame Enabled {
          }
        }
        n2913 = case shown="True" "OK Button 17" {
          frame False {
          }
          frame True {
            (unwired) 0  # existing file
            w4105 = "Choose a datalog file to open"  # prompt
            n2914 = local write "OK Button 17"(FALSE ("OK Button 17")) -> ()
            n2915 = local read "String"() -> (w4100:string)
            n2916 = String To Path(string=w4100) -> (path=w4101:path)
            n2917 = File Dialog(6:"*.duf" ("pattern"), 7:w4105, 11:w4101) -> (0:w4092:errorcluster, 3:w4111:path)  [unwired: 4 in, 2 out]
            n2918 = Unbundle(w4092) -> ()  [unwired: 3 out]
            n2919 = Open/Create/Replace File "Open File"(file path (use dialog)=w4111) -> (refnum out=w4103:refnum<file>)  [unwired: 5 in, 2 out]
            n2920 = Strip Path(path=w4111) -> (name=w4109:string)  [unwired: 1 out]
            n2921 = Path To String(path=w4111) -> (string=w4094:string)
            n2922 = while {
              tunnel: w4103 -> [w4115]
              i -> [w4112]
              stop <- w4113 continue-if-true
              (unwired) TRUE ("line mode (F)")
              n2923 = Read from Text File "Read File"(file (use dialog)=w4115) -> (text=w4114:string)  [unwired: 3 in, 3 out]
              n2924 = local write "Numeric 16"(w4112) -> ()
              n2925 = String Length(string=w4114) -> (length=w4117:i32)
